vi "Composed State to Default.vi"(8 "error in (no error)":errorcluster, 11 "Context in":refnum<class "State Pattern.lvclass">) -> (0 "error out":errorcluster, 3 "Context out":refnum<class "State Pattern.lvclass">)   [LabVIEW 2021, in "State Pattern.lvclass"]
uses:
  State Pattern.lvclass
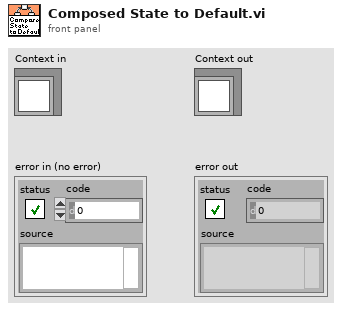
[diagram p1: front panel]
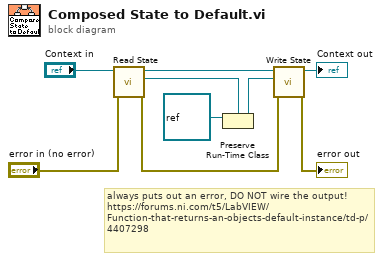
[diagram p0: block diagram]
diagram:
  # "always puts out an error, DO NOT wire the output!\nhttps://forums.ni.com/t5/LabVIEW/Function-that-returns-an-objects-default-instance/td-p/4407298"
  n1 = call-dynamic "Read State.vi"("error in"="error in (no error)", "Context in"="Context in") -> ("error out"=w8:errorcluster, "State"=w2:refnum<class "State Pattern.lvclass">, "Context out"=w9:refnum<class "State Pattern.lvclass">)  [unwired: 7 in]
  n2 = Preserve Run-Time Class(object in=refnum<class> refnum ("LabVIEW Object"), 2:w2) -> (object out=w1:refnum<class "State Pattern.lvclass">)  [unwired: 1 in, 1 out]
  n3 = call-dynamic "Write State.vi"("error in"=w8, "State"=w1, "Context in"=w9) -> ("error out"=→"error out":errorcluster, "Context out"=→"Context out":refnum<class "State Pattern.lvclass">)  [unwired: 7 in]
